vi "LitePoint_VSGConfig_PowerFreq.vi"(8 "error in (no error)":errorcluster, 9 "Power":dbl, 10 "Freq_MHz":dbl=3500.0, 11 "VISA resource name":refnum<visa-resource-name>="LitePoint_IQxstream") -> (0 "error out":errorcluster, 3 "VISA resource name out":refnum<visa-resource-name>="LitePoint_IQxstream")   [LabVIEW 2020, in "LitePoints.lvlib"]
uses:
  LitePoints.lvlib
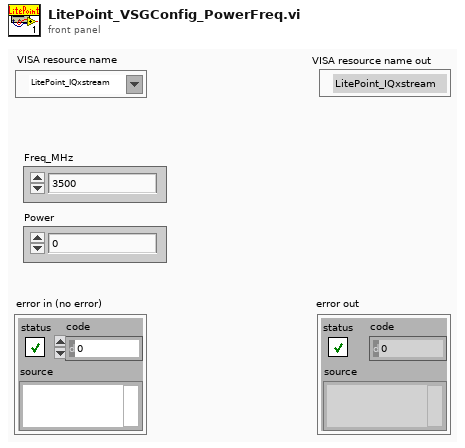
[diagram p1: front panel]
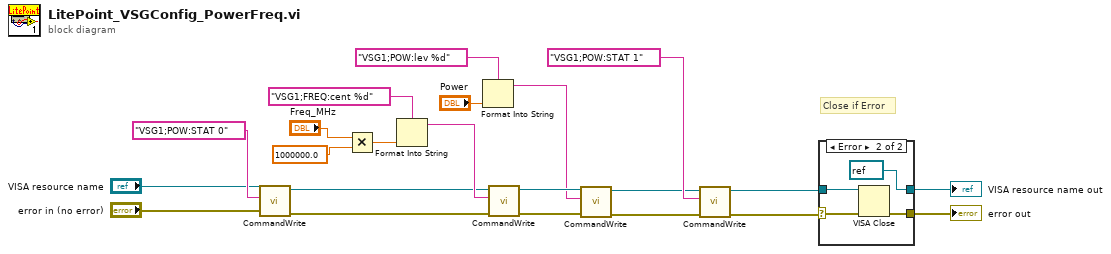
[diagram p0: block diagram]
diagram:
  # "Close if Error"
  n1 = call "CommandWrite.vi"("error in (no error)"="error in (no error)", "Write Buffer"="VSG1;POW:STAT 0", "VISA resource name"="VISA resource name") -> ("error out"=w3:errorcluster, "VISA resource name out"=w4:refnum<visa-resource-name>)  [unwired: 7 in]
  n2 = Multiply(x="Freq_MHz", y=1000000.0) -> (x*y=w13:dbl)
  n3 = Format Into String(format string="VSG1;FREQ:cent %d", w13) -> (resulting string=w14:string)  [unwired: 2 in, 1 out]
  n4 = Format Into String(format string="VSG1;POW:lev %d", "Power") -> (resulting string=w16:string)  [unwired: 2 in, 1 out]
  n5 = call "CommandWrite.vi"("error in (no error)"=w3, "Write Buffer"=w14, "VISA resource name"=w4) -> ("error out"=w19:errorcluster, "VISA resource name out"=w20:refnum<visa-resource-name>)  [unwired: 7 in]
  n6 = call "CommandWrite.vi"("error in (no error)"=w19, "Write Buffer"=w16, "VISA resource name"=w20) -> ("error out"=w1:errorcluster, "VISA resource name out"=w2:refnum<visa-resource-name>)  [unwired: 7 in]
  n7 = call "CommandWrite.vi"("error in (no error)"=w1, "Write Buffer"="VSG1;POW:STAT 1", "VISA resource name"=w2) -> ("error out"=w7:errorcluster, "VISA resource name out"=w8:refnum<visa-resource-name>)  [unwired: 7 in]
  n8 = case shown="Error" w7 {
    selector: w7 -> [w23 w26]
    tunnel: w8 -> [w24 w27]
    tunnel: [w24 refnum<visa-resource-name> refnum ("VISA resource name out")] -> w22
    tunnel: [w23 w25] -> w21
    frame No Error {
    }
    frame Error {
      n9 = VISA Close(VISA resource name=w27, error in (no error)=w26) -> (error out=w25:errorcluster)
    }
  }
  "VISA resource name out" <- w22
  "error out" <- w21
